vi "Joystick 2 ColorWheel.vi"(8 "Secondary Joystick Values":dbl[](array[numeric]), 11 "Secondary Joystick Buttons":bool[](array[boolean])) -> (3 "SpinnerActions":T1)   [LabVIEW 2019]
uses:
  Controls/Spinner Actions.ctl
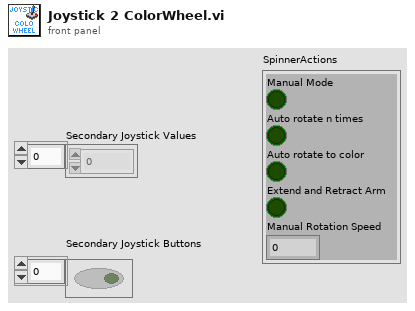
[diagram p1: front panel]
types:
  T1 = typedef "Spinner Actions.ctl" = cluster{"Manual Mode ":bool, "Auto rotate n times":bool, "Auto rotate to color\t":bool, "Extend and Retract Arm\t":bool, "Manual Rotation Speed":dbl}
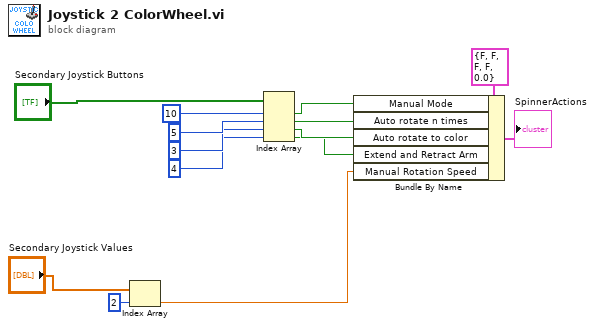
[diagram p0: block diagram]
diagram:
  n1 = Index Array(array="Secondary Joystick Values", index=2) -> (element=w3:dbl)
  n2 = Index Array(array="Secondary Joystick Buttons", index #1=10 ("index"), index #2=5 ("index"), index #3=3 ("index"), index #4=4 ("index")) -> (element #1=w12:bool, element #2=w11:bool, element #3=w2:bool, element #4=w1:bool)
  n3 = Bundle By Name(cluster=T1 {"Manual Mode "=FALSE, "Auto rotate n times"=FALSE, "Auto rotate to color\t"=FALSE, "Extend and Retract Arm\t"=FALSE, "Manual Rotation Speed"=0.0} ("SpinnerActions"), "Manual Mode"=w12, "Auto rotate n times"=w11, "Auto rotate to color"=w2, "Extend and Retract Arm"=w1, "Manual Rotation Speed"=w3) -> (→"SpinnerActions":T1)
